vi "strGlobalVariable.vi"() -> ()   [LabVIEW 2011]
panel:
  in  "strWWSetProgress_Step":T1={"enumRunningProgress"=enum."PROGRESS_INITIAL", "enumRunMode"=enum."RUNMODE_READY", "enumPowerState"=enum."POWER_STATE_POWER_OFF", "strWWStep"={"enumInitProgressStep"=enum."INIT_PROGRESS_INIT", "enumPreWashStep"=enum."PREWASH_INIT", "enumWashStep"=enum."WASH_INIT", "enumRinseStep"=enum."RINSE_INIT", "enumFinalSpinStep"=enum."FINALSPIN_INIT", "enumFinishStep"=enum."FINISH_STEPORDER_COUNT_INFORMATION_SAVE"}}
  out "mu08CmdArray":u8[][](array[numeric])=[[90, 165, 6, 127, 3, 0, 0, 0, 133, 0], [90, 165, 10, 240, 1, 0, 251, 2, 247, 23], [90, 165, 10, 240, 1, 0, 251, 4, 151, 209], [90, 165, 10, 240, 1, 0, 251, 6, 183, 147], [90, 165, 8, 1, 240, 0, 80, 135, 0, 0]] format="0x%x"
  in  "enumWDCourse":T2(ring)
  in  "WW_ParameterData":T3(ring)
  in  "enumCourse":T4(ring)
  out "StrArrayConstant":string[](array[string])=["ValveCold", "ValveHot", "ValvePre", "WaterShot", "ValveBleach", "ValveDry", "ValveMist", "ValveSteam", "ValveChange", "ValveSoftener", "ValveFilter", "ValveActiveWash", "ValveHotActiveWash", "MotorAC", "MotorFan", "MotorClutch", "DoorLock", "MotorAutoDetergent", "MotorAutoRinse", "SSR", "MainRelay", "PumpDrain", "PumpCircuration", "PumpBubble", "MotorDistributor", "TurbiditySensorOnOff", "ActuatorDry", "ActuatorDoorOpen", "VaneCW", "VaneCCW", "IVTPower1", "IVTPower2", "HeaterWash", "HeaterDry", "HeaterSteam", "HeaterDryerLarge", "HeaterDryerSmall", "Motor CW", "Motor CCW", "MotorDirection", "IsDoubleDoorOpen", "IsDoubleDoorOpenLock", "WaterLevel", "WaterTemp", "AirTemp", "IPMTemp", "MotorActualRPM", "MotorTargetRPM", "FanActualRPM", "FanTargetRPM", "MemsSensorA", "MemsSensorB", "MemsSensorC", "TouchSensor", "WaterThermistorADC", "LeakageSensor", "DCLink", "IsDoorOpen", "IsTimeShort", "Progress", "Step", "TotalRemainTime", "StepRemainTime", "WeightSensingLowData", "WeightSensingResult", "RunState", "PowerState", "SoundID", "ErrorCode", "OptionData", "VersionMain", "VersionSub", "VersionInverter", "VersionTouch", "RequestUIData", "RequestSensorData", "RequestVersionData", "IsConnectedHASS", "RequestWMInfoData", "RequestWMTestData", "CommandRx"]
  out "strResultArrayOut_4ed":string[](array[string])
  out "strResultArrayOut_3rd":string[](array[string])
  out "strResultArrayOut_2nd":string[](array[string])
  out "strResultArrayOut_1st":string[](array[string])
  # "进入DFTP模式"
  # "接收Sensor Data"
  # "接收Version Data"
  # "接收Sensor+Version Data"
  # "请求接收数据信息"
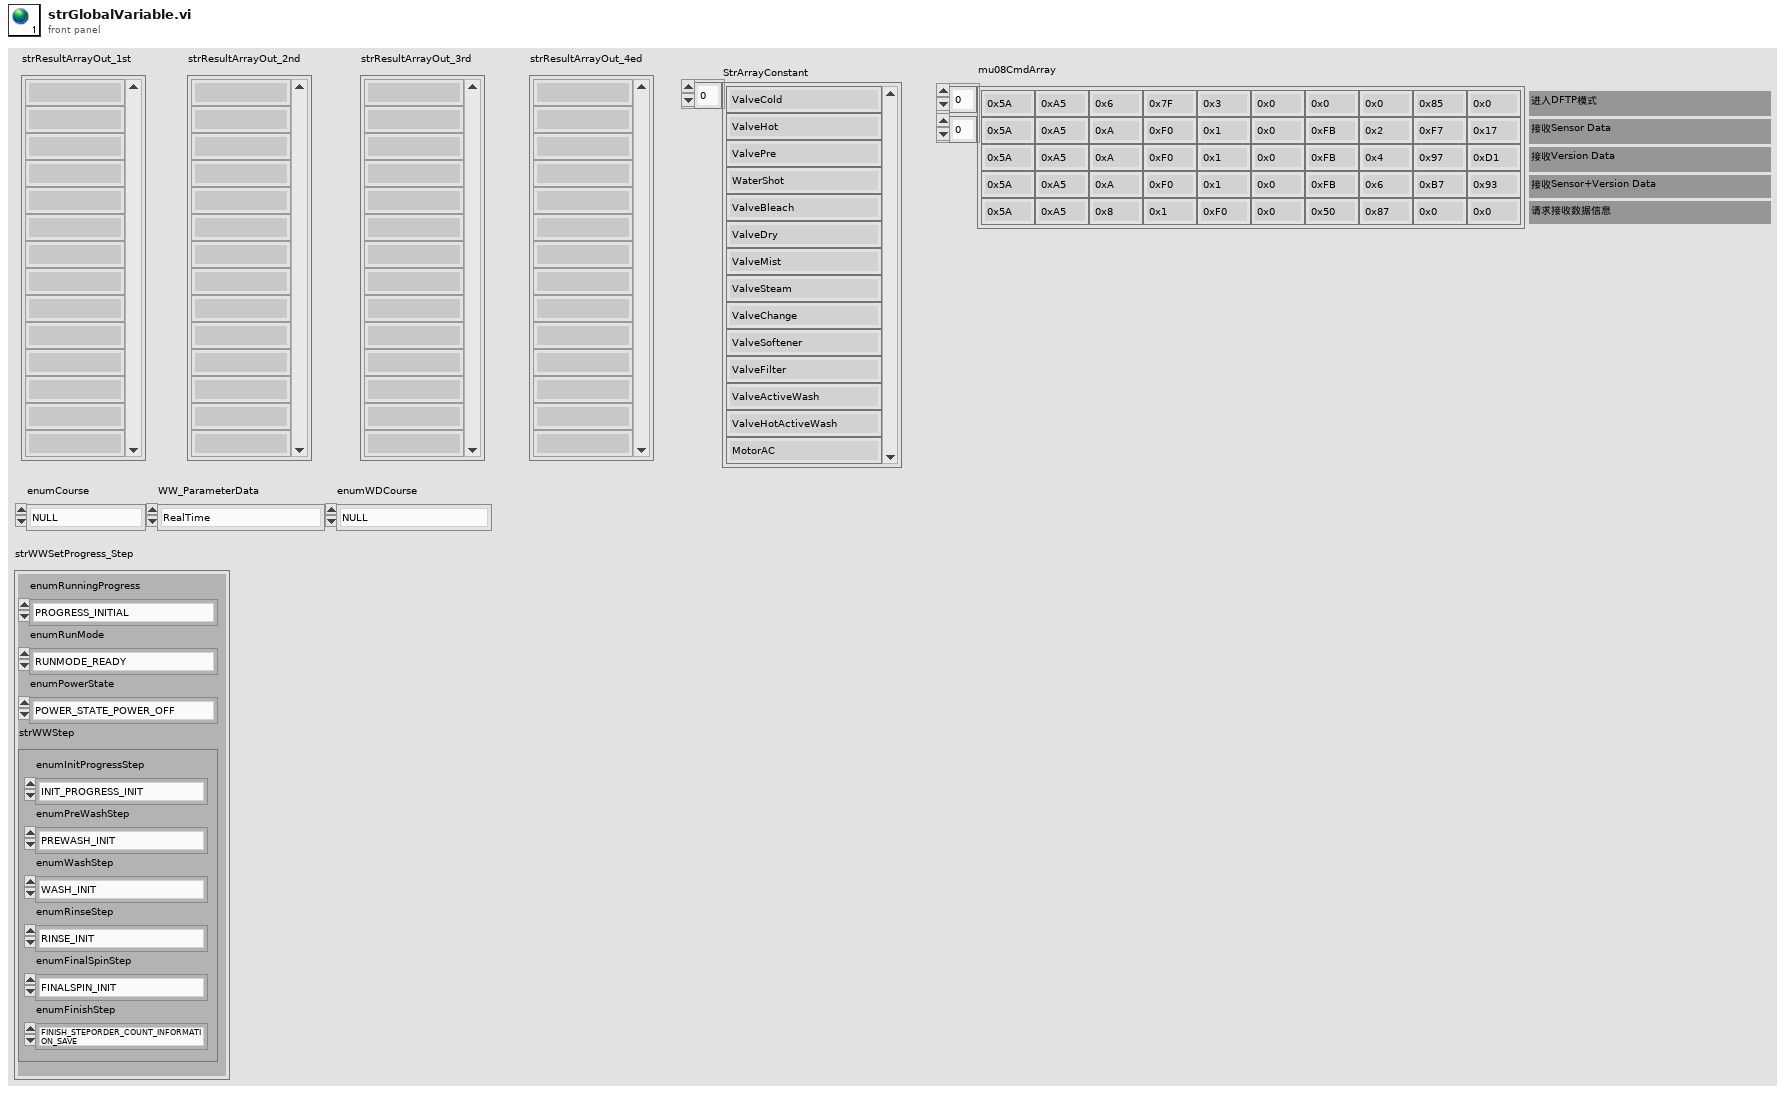
[diagram p1: front panel]
types:
  T1 = cluster{"enumRunningProgress":enum16{"PROGRESS_INITIAL", "PROGRESS_RESERVE", "PROGRESS_PREWASH", "PROGRESS_WASH", "PROGRESS_RINSE", "PROGRESS_FINALSPIN", "PROGRESS_DRY", "PROGRESS_AIRWASH", "PROGRESS_FINISH", "PROGRESS_END", "PROGRESS_MAX"}, "enumRunMode":enum16{"RUNMODE_CHECK_READY_HOT_CONDITION_AND_PROCESS", "RUNMODE_READY", "RUNMODE_READY_LAUNDARYADD", "RUNMODE_START_INITIAL", "RUNMODE_DOOR_SAFETY", "RUNMODE_START_DOORLOCK_CHK", "RUNMODE_CHECK_START_HOT_CONDITION_AND_PROCESS", "RUNMODE_RUNNING", "RUNMODE_PAUSE_INITIAL", "RUNMODE_PAUSE_CHECK_MOTOR_STOP", "RUNMODE_PAUSE_HOT_WARNING", "RUNMODE_PAUSE_LAUNDARYADD_AND_DOOR_UNLOCK", "RUNMODE_PAUSE_PAUSED_STEP", "RUNMODE_RESUME_INITIAL_STEP"}, "enumPowerState":enum16{"POWER_STATE_POWER_OFF", "POWER_STATE_POWER_UP_INIT", "POWER_STATE_POWER_UP_START", "POWER_STATE_POWER_UP_DONE", "POWER_STATE_POWER_ON", "POWER_STATE_POWER_DOWN", "POWER_STATE_POWER_OFF_FOR_OTN", "POWER_STATE_POWER_SLEEP_MODE"}, "strWWStep":cluster{"enumInitProgressStep":enum16{"INIT_PROGRESS_INIT", "INIT_PROGRESS_FIRST_DRAIN_INITIAL", "INIT_PROGRESS_FIRST_DRAIN"}, "enumPreWashStep":enum16{"PREWASH_INIT", "PREWASH_WEIGHT", "PREWASH_WATERSUPPLY", "PREWASH_WASH1", "PREWASH_WASH2", "PREWASH_DRAIN", "PREWASH_SPIN", "PREWASH_END"}, "enumWashStep":enum16{"WASH_INIT", "WASH_DRUMWASHWATER", "WASH_DRUMWASHRINSE", "WASH_DRUMWASHDRAIN", "WASH_WEIGHT", "WASH_DRUMWASHWEIGHT", "WASH_WATERSUPPLY", "WASH_WASH1", "WASH_WASH2", "WASH_WASH3", "WASH_WASH4", "WASH_WASH5", "WASH_WASH6", "WASH_MAGICSTEAM_DRAIN", "WASH_MAGICSTEAM_SUPPLY", "WASH_MAGICSTEAM_TUMBLE", "WASH_END"}, "enumRinseStep":enum16{"RINSE_INIT", "RINSE_DRAIN", "RINSE_SUDS_REDUCTION", "RINSE_SPIN", "RINSE_WATERSUPPLY", "RINSE_RINSE", "RINSE_REMOVE_SUDS", "RINSE_END"}, "enumFinalSpinStep":enum16{"FINALSPIN_INIT", "FINALSPIN_DRAIN", "FINALSPIN_SUDS_REDUCTION", "FINALSPIN_SPIN", "FINALSPIN_LOOSE", "FINALSPIN_END"}, "enumFinishStep":enum16{"FINISH_STEPORDER_COUNT_INFORMATION_SAVE", "FINISH_STEPORDER_ENDSOUND_PLAY", "FINISH_STEPORDER_UNLOCK_CHECK", "FINISH_STEPORDER_AGING_WAITTIME_CHECK", "FINISH_STEPORDER_AGING_WAITTING", "FINISH_STEPORDER_NOMAL_WAITTING", "FINISH_STEPORDER_DRUMLIGHT_CHECK", "FINISH_STEPORDER_CHECK_MOTOR_STOP", "FINISH_STEPORDER_CHILDLOCK_WAITTING", "FINISH_STEPORDER_CLOSE"}}}
  T2 = enum16{"NULL", "Cotton", "Synthetics", "Wool", "BabyCare", "OutDoorCare", "RinseSpin", "EcoDrumClean", "DailyWash", "QuikWash", "SuperEcoWash", "SyntheticsDry", "CottonDry", "Sanitization", "Deodorization"}
  T3 = enum16{"RealTime", "WaterLevel", "WaterTemp", "AirTemp", "IPMTemp", "MotorActualRPM", "MotorTargetRPM", "FanActualRPM", "MemsSensorA", "MemsSensorB", "MemsSensorC", "WaterThermistorADC", "TouchSensor", "LeakageSensor", "DCLink", "IsDoorOpen", "IsTimeShort", "Progress", "Step", "TotalRemainTime", "StepRemainTime", "WeightSensingLowData", "WeightSensingResult", "ColdValve", "HotValve", "PreValve", "WaterShotValve", "BleachValve", "DryValve", "SteamValve", "SoftenerValve", "FilterValve", "IsDoorLocked", "SSRCommon", "MainRelay", "ACTUATOR2", "WaterDrainer", "CirculationPump", "WaterHeater", "DryHeater", "SteamHeater", "MotorDriveDirection", "IsDoubleDoorOpen", "IsDoubleDoorLock", "RunStateID", "PowerStateID", "SoundID", "ErrorCode", "OptionData", "MainVersion", "SUBVersion", "InverterVersion"}
  T4 = enum8{"NULL", "Course", "eCotton", "Synthetics", "Wool", "Spin", "RinseSpin", "EcoDrumClean", "DarkGarment", "OutDoorCare", "BabyCare", "Delicates", "Bedding", "SuperEcoWash", "SuperSpeed"}
diagram:
